vi "Call NIPKG CLI (runas admin).vi"(8 "error in (no error)":errorcluster, 11 "command":string) -> (0 "error out":errorcluster)   [LabVIEW 2014, in "NIPM_API.lvlib"]
doc: "This VI calls the nipkg.exe command-line interface (CLI) from the command line as an admin.\n\nNotes:\nThis VI will launch a Windows dialog asking for permission to run and requires the user to have admin rights. This VI uses the ShellExecuteA function in <system32>\\shell32.dll.\n\nThis VI will not return an error if the nipkg command failed. This VI only returns an error if the ShellExecuteA function itself has an error.\n\nINPUT(s)\n<B>Command</B> is a string containing the specific nipkg CLI command (e.g. install, remove) to execute as an admin."
uses:
  NIPM_API.lvlib
  <vilib>/Utility/sysdir.llb/System Directory Type.ctl
panel:
  out "HINSTANCE":i32
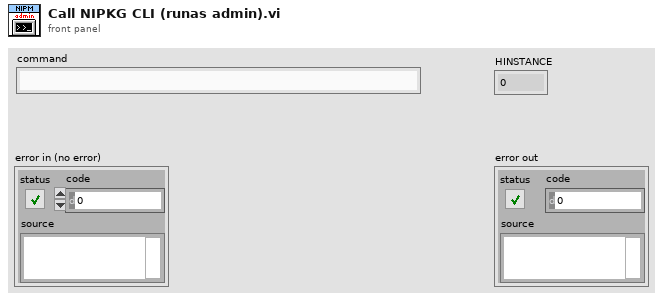
[diagram p1: front panel]
types:
  T1 = typedef "System Directory Type.ctl" = i32
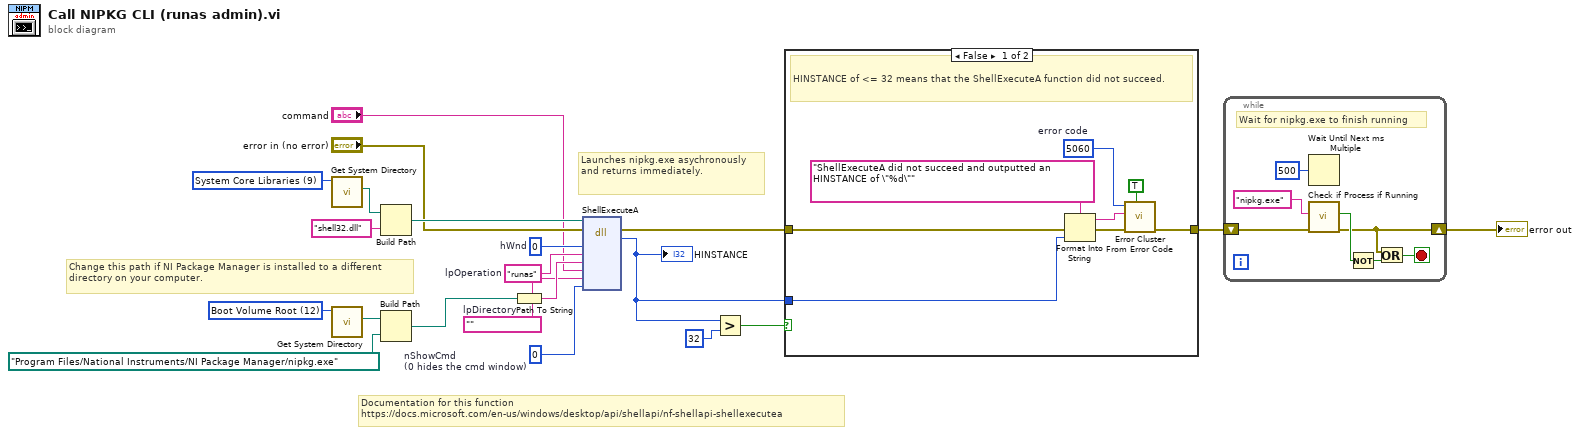
[diagram p0: block diagram]
diagram:
  w7 = 0  # nShowCmd (0 hides the cmd window)
  w8 = ""  # lpDirectory
  w12 = "runas"  # lpOperation
  w13 = 0  # hWnd
  w18 = T1 9 items=["User Home"=0, "User Desktop"=1, "User Documents"=2, "User Application Data"=3, "User Preferences"=4, "User Temporary"=5, "Public Documents"=6, "Public Application Data"=7, "Public Preferences"=8, "Public Cache"=13, "System Core Libraries"=9, "System Installed Libraries"=10, "Application Files"=11, "Boot Volume Root"=12] ("system directory type")
  w19 = T1 12 items=["User Home"=0, "User Desktop"=1, "User Documents"=2, "User Application Data"=3, "User Preferences"=4, "User Temporary"=5, "Public Documents"=6, "Public Application Data"=7, "Public Preferences"=8, "Public Cache"=13, "System Core Libraries"=9, "System Installed Libraries"=10, "Application Files"=11, "Boot Volume Root"=12] ("system directory type")
  # "Launches nipkg.exe asychronously and returns immediately."
  # "Documentation for this function\nhttps://docs.microsoft.com/en-us/windows/desktop/api/shellapi/nf-shellapi-shellexecutea"
  # "Change this path if NI Package Manager is installed to a different directory on your computer."
  n1 = call <vilib>:"Get System Directory.vi"("system directory type"=w18) -> ("system directory"=w17:path)  [unwired: 10 in]
  n2 = call <vilib>:"Get System Directory.vi"("system directory type"=w19) -> ("system directory"=w20:path)  [unwired: 10 in]
  n3 = Build Path(base path=w17, name or relative path="shell32.dll") -> (appended path=w15:path)
  n4 = Build Path(base path=w20, name or relative path=path "Program Files/National Instruments/NI Package Manager/nipkg.exe" ("working directory")) -> (appended path=w14:path)
  n5 = Path To String(path=w14) -> (string=w11:string)
  n6 = dll-call lib="C:/Windows/System32/shell32.dll" fn="ShellExecuteA"(path in=w15, error in="error in (no error)", "hWnd"=w13, "lpOperation"=w12, "lpFile"=w11, "lpParameters"="command", "lpDirectory"=w8, "nShowCmd"=w7) -> (error out=w4:errorcluster, "HINSTANCE"=w3:i32)  [unwired: 7 in, 1 out]
  "HINSTANCE" <- w3
  n7 = Greater?(x=w3, y=32) -> (0:w5:bool)
  n8 = case shown="False" w5 {
    tunnel: w4 -> [w24 w30]
    tunnel: [w27 w30] -> w2
    tunnel: w3 -> [w25 _]
    frame False {
      w28 = 5060  # error code
      # "HINSTANCE of <= 32 means that the ShellExecuteA function did not succeed."
      n9 = Format Into String(format string="ShellExecuteA did not succeed and outputted an HINSTANCE of \"%d\"" ("error message (\"\")"), error in=w24, w25) -> (resulting string=w22:string, error out=w23:errorcluster)  [unwired: 1 in]
      n10 = call <vilib>:"Error Cluster From Error Code.vi"("show call chain? (False)"=TRUE, "error in (no error)"=w23, "error message (\"\")"=w22, "error code (0)"=w28) -> ("error out"=w27:errorcluster)  [unwired: 5 in]
    }
    frame True {
      # "ShellExecuteA did not return an error"
    }
  }
  n11 = while {
    shift-right: [w32] -> w1
    shift-left: w2 -> [w36]
    stop <- w31 stop-if-true
    # "Wait for nipkg.exe to finish running"
    # "Wait for nipkg.exe to finish running"
    n12 = Wait Until Next ms Multiple(millisecond multiple=u32 500) -> ()  [unwired: 1 out]
    n13 = call "Check if Process if Running.vi"("error in (no error)"=w36, "Process Name"="nipkg.exe") -> ("error out"=w32:errorcluster, "Running?"=w35:bool)  [unwired: 8 in]
    n14 = Not(x=w35) -> (.not. x?=w33:bool)
    n15 = Or(x=w32, y=w33) -> (x .or. y?=w31:bool)
  }
  "error out" <- w1
